vi "Manage Modules.vi"() -> (12 "Cancelled?":bool, 14 "Selected Modules":string[](array[string]), 15 "Modules Refs":refnum<vi>[](array[refnum]))   [LabVIEW 2019]
panel:
  in  "Cancel":bool
  in  "OK":bool
  in  "Modules Manager":cluster{"Name":string, "Check":bool}[](array[cluster])
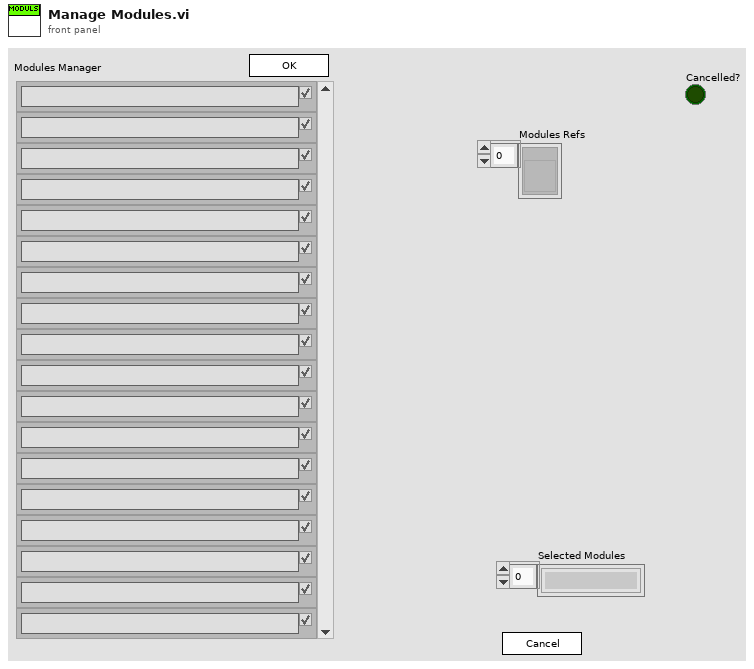
[diagram p1: front panel]
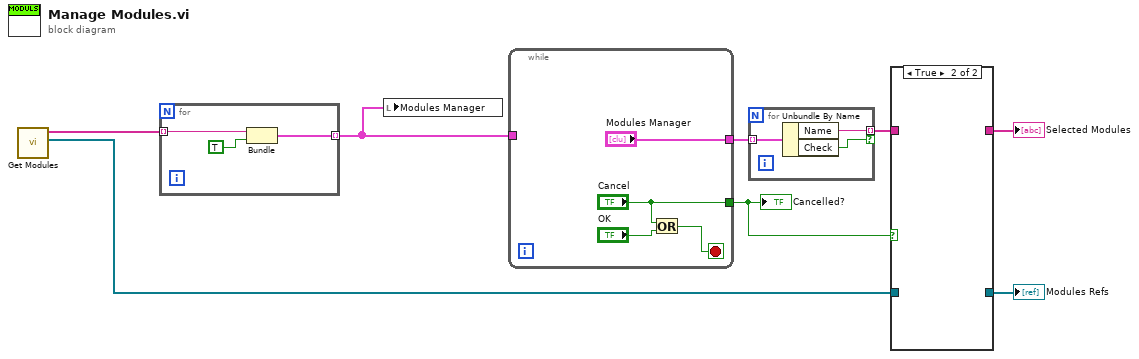
[diagram p0: block diagram]
diagram:
  n1 = call "Get Modules.vi"() -> ("Modules Refs"=w5:refnum<vi>[], "Modules Names"=w6:string[])  [unwired: 8 in, 2 out]
  n2 = for {
    tunnel: w6 -> [w11] mode=indexing
    tunnel: [w9] -> w7 mode=indexing
    n3 = Bundle("Name"=w11, TRUE) -> (w9:cluster{"Name":string, bool})  [unwired: 1 in]
  }
  n4 = local write "Modules Manager"(w7) -> ()
  n5 = while {
    tunnel: ["Cancel"] -> w1
    tunnel: ["Modules Manager"] -> w8
    tunnel: w7 -> [_]
    stop <- w14 stop-if-true
    n6 = Or(x="Cancel", y="OK") -> (x .or. y?=w14:bool)
  }
  "Cancelled?" <- w1
  n7 = for {
    tunnel: w8 -> [w18] mode=indexing
    tunnel: [w17] -> w2 mode=indexing if=w16
    n8 = Unbundle By Name(w18) -> ("Name"=w17:string, "Check"=w16:bool)
  }
  n9 = case shown="True" w1 {
    tunnel: [w20 _] -> w4
    tunnel: w5 -> [w20 _]
    tunnel: [w19 _] -> w3
    tunnel: w2 -> [w19 _]
    frame False {
    }
    frame True {
    }
  }
  "Selected Modules" <- w3
  "Modules Refs" <- w4
